vi "Byte Buffer.Get pointers.vi"(8 "error in (no error)":errorcluster, 11 "Byte Buffer in":refnum<class "Byte Buffer.lvclass">) -> (0 "error out":errorcluster, 2 "Byte Buffer pointers":T1, 3 "Byte Buffer out":refnum<class "Byte Buffer.lvclass">)   [LabVIEW 2016, in "VeriStand Data.lvlib" / "Byte Buffer.lvclass"]
uses:
  Byte Buffer.lvclass
  Byte Buffer.Pointers.ctl
  Byte Buffer.lvclass/Byte Buffer.ctl
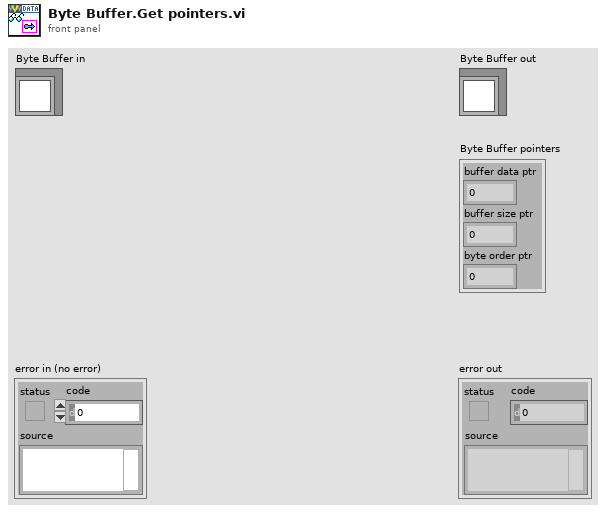
[diagram p1: front panel]
types:
  T1 = typedef "VeriStand Data.lvlib/Byte Buffer.lvclass/Byte Buffer.Pointers.ctl" = cluster{"buffer data ptr":u64, "buffer size ptr":u64, "byte order ptr":u64}
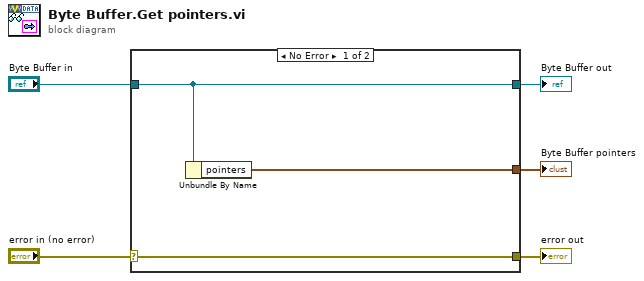
[diagram p0: block diagram]
diagram:
  n1 = case shown="No Error" "error in (no error)" {
    selector: "error in (no error)" -> [w8 w9]
    tunnel: [w8 w9] -> w4
    tunnel: [w7 w10] -> w2
    tunnel: "Byte Buffer in" -> [w7 w10]
    tunnel: [w6 _] -> w1
    frame No Error {
      n2 = Unbundle By Name(w7) -> ("pointers"=w6:T1)
    }
    frame Error {
    }
  }
  "error out" <- w4
  "Byte Buffer out" <- w2
  "Byte Buffer pointers" <- w1
